vi "EEI EXP9.vi"() -> ()   [LabVIEW 2020]
uses:
  <vilib>/numeric/Random Number (Range) U64.vi
  <vilib>/numeric/sub_Random U32.vi
panel:
  in  "y":dbl
  in  "x":dbl
  out "x^2":dbl
  out "Waveform Graph":u64[](graph)
  out "Waveform Chart":u64[](graph)
  out "Array":u64[](array[numeric])
  out "current time":timestamp
  out "x^2":dbl
  in  "y":dbl
  in  "x":dbl
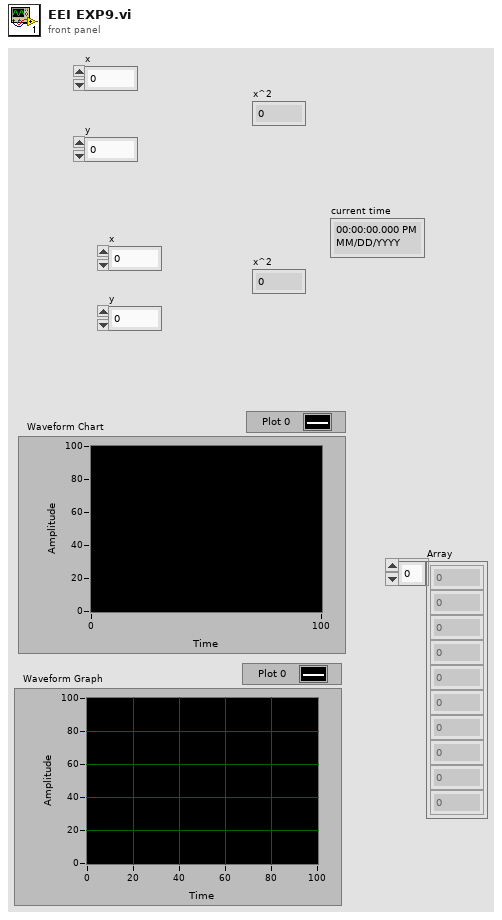
[diagram p1: front panel]
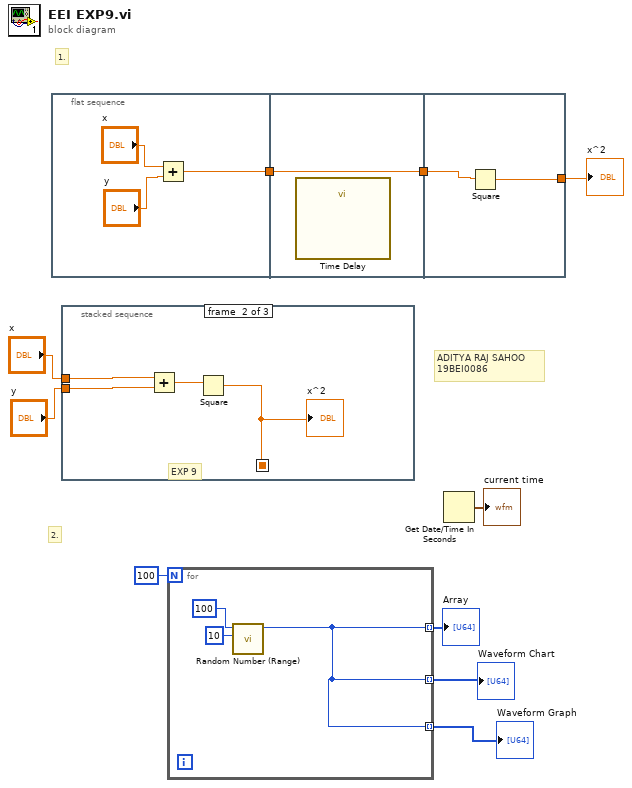
[diagram p0: block diagram]
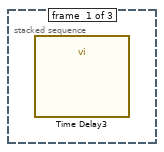
[diagram p2: hidden frame]
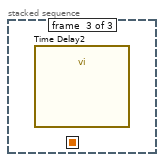
[diagram p3: hidden frame]
diagram:
  # "2."
  # "1."
  # "ADITYA RAJ SAHOO\n19BEI0086"
  # "EXP 9"
  n1 = flat-sequence {
    tunnel: [w11] -> w10
    tunnel: w10 -> [w14]
    tunnel: [w14] -> w8
    tunnel: [w16] -> w9
    tunnel: w8 -> [w15]
    frame #0 {
      n2 = Add(x="x", y="y") -> (x+y=w11:dbl)
    }
    frame #1 {
      n3 = call "Time Delay"() -> ()  [unwired: 11 in, 1 out]
    }
    frame #2 {
      n4 = Square(x=w15) -> (x^2=w16:dbl)
    }
  }
  n5 = stacked-sequence {
    seq-local: [_ w17 _] -> [_ _ _]
    tunnel: "y" -> [_ w20 _]
    tunnel: "x" -> [_ w19 _]
    frame #0 {
      n6 = call "Time Delay3"() -> ()  [unwired: 11 in, 1 out]
    }
    frame #1 {
      n7 = Add(x=w19, y=w20) -> (x+y=w18:dbl)
      n8 = Square(x=w18) -> (x^2=w17:dbl)
      "x^2" <- w17
    }
    frame #2 {
      n9 = call "Time Delay2"() -> ()  [unwired: 11 in, 1 out]
    }
  }
  n10 = for {
    N: 100 -> [_]
    tunnel: [w21] -> w5 mode=indexing
    tunnel: [w21] -> w4 mode=indexing
    tunnel: [w21] -> w3 mode=indexing
    n11 = call-poly <vilib>:"Random Number (Range).vi"("lower bound (0)"=u64 10, "upper bound (100)"=u64 100) -> ("number"=w21:u64)  [unwired: 9 in]
  }
  "Array" <- w5
  "Waveform Chart" <- w4
  "Waveform Graph" <- w3
  n12 = Get Date/Time In Seconds() -> (seconds since 1Jan1904=→"current time":timestamp)
  "x^2" <- w9
